vi "Threshold Detector Comparison.vi"() -> ()   [LabVIEW 2023]
doc: "Uses the Advanced Threshold Peak Detector PtByPt VI to analyze the input data sequence for valid peaks. The example keeps a count of the number of peaks encountered and a record of indices, which locates the points that exceed the threshold value in a valid peak."
uses:
  <vilib>/Analysis/1siggen.llb/Ramp Pattern by Samples.vi
  <vilib>/ptbypt/NI_PtbyPt.lvlib
  <vilib>/Analysis/NI_AALPro.lvlib
  <vilib>/Analysis/NI_AALBase.lvlib
panel:
  out "number of crossings":i32
  in  "Stop":bool
  out "index":i32
  out "detected":bool
  out "Array-based results":T1(graph)
  in  "Threshold":dbl(slide)=18.367346938775512 scale=-60.0..60.0
  out "Indices":i32[](array[numeric])
  in  "Width":i32(slide)=1 scale=0.0..20.0
  in  "initialize":bool
  # "Overview: Uses the Threshold Peak Detector PtByPt VI to analyze data for valid peaks.\nRequirements: LabVIEW Full Development System\nInstructions: \n1. Run the VI.\n2. Change the Threshold value and verify that peaks are not detected when the threshold is above the signal amplitude.\n3. Change the Width value and observe the effects on the results.\n4. Click Stop to stop the VI."
  # "Array-based results"
  # "Point-by-point results"
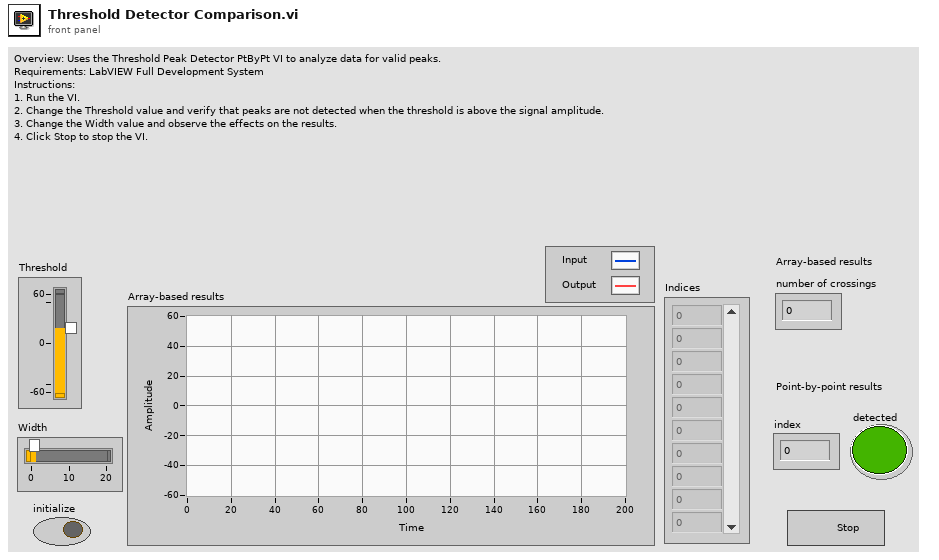
[diagram p1: front panel]
types:
  T1 = cluster{"Current Queue":dbl[], "Current Queue":dbl[]}[]
  T2 = cluster{"Ramp Pattern":dbl[], "Current Queue":dbl[]}
  T3 = cluster{"Ramp Pattern":dbl[], "Current Queue":dbl[]}[]
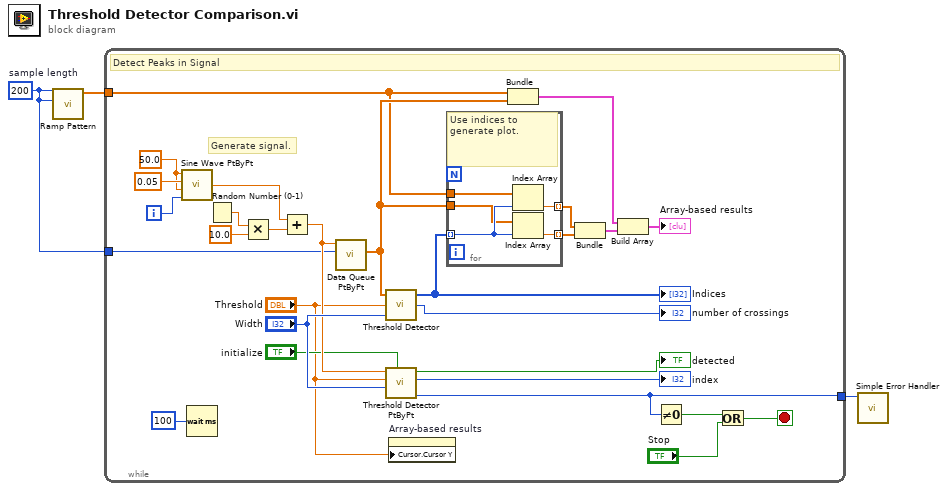
[diagram p0: block diagram]
diagram:
  w2 = 200  # sample length
  n1 = call-poly <vilib>:"Ramp Pattern.vi"("end"=w2, "samples"=w2) -> ("Ramp Pattern"=w3:dbl[])  [unwired: 8 in, 1 out]
  n2 = while {
    tunnel: w3 -> [w15]
    tunnel: w2 -> [w10]
    tunnel: [w6] -> w1
    i -> [w12]
    stop <- w29 stop-if-true
    w5 = 50.0 ("amplitude")
    # "Generate signal."
    # "Detect Peaks in Signal"
    n3 = call <vilib>:"Sine Wave PtByPt.vi"("time"=w12, "phase"=w5, "frequency"=0.05, "amplitude"=w5) -> ("sine wave"=w8:dbl)
    n4 = Wait (ms)(milliseconds to wait=u32 100) -> ()  [unwired: 1 out]
    n5 = Random Number (0-1)() -> (number: 0 to 1=w31:dbl)
    n6 = Multiply(x=w31, y=10.0) -> (x*y=w23:dbl)
    n7 = Add(x=w8, y=w23) -> (x+y=w14:dbl)
    n8 = call <vilib>:"Data Queue PtByPt.vi"("sample length"=w10, "input data point"=w14) -> ("Current Queue"=w18:dbl[])  [unwired: 5 in, 4 out]
    n9 = call <vilib>:"Threshold Detector.vi"("width"="Width", "threshold"="Threshold", "X"=w18) -> ("count"=→"number of crossings":i32, "Indices"=w16:i32[])  [unwired: 1 out]
    "Indices" <- w16
    n10 = call <vilib>:"Threshold Detector PtByPt.vi"("initialize"="initialize", "width"="Width", "threshold"="Threshold", "x"=w14) -> ("error"=w6:i32, "index"=→"index":i32, "detected"=→"detected":bool)  [unwired: 5 in]
    n11 = property on="Array-based results" class="XYGraph (strict)"("Cursor.Cursor Y"="Threshold") -> ()  [unwired: 2 in, 2 out]
    n12 = for {
      tunnel: w15 -> [w35]
      tunnel: w18 -> [w34]
      tunnel: w16 -> [w36] mode=indexing
      tunnel: [w33] -> w26 mode=indexing
      tunnel: [w32] -> w25 mode=indexing
      # "Use indices to generate plot."
      n13 = Index Array(array=w35, index=w36) -> (element=w33:dbl)
      n14 = Index Array(array=w34, index=w36) -> (element=w32:dbl)
    }
    n15 = Bundle("Ramp Pattern"=w15, "Current Queue"=w18) -> (w28:T2)  [unwired: 1 in]
    n16 = Bundle(w26, w25) -> (w24:cluster{dbl[], dbl[]})  [unwired: 1 in]
    n17 = Build Array(w28, w24) -> (→"Array-based results":T3)
    n18 = Not Equal To 0?(x=w6) -> (x != 0?=w30:bool)
    n19 = Or(x=w30, y="Stop") -> (x .or. y?=w29:bool)
  }
  n20 = call <vilib>:"Simple Error Handler.vi"("error code (no error:0)"=w1) -> ()  [unwired: 4 in, 5 out]
